vi "STEPkgDriver_LINC_Server.vi"() -> ()   [LabVIEW 2018, in "STEPkgDriver_LINC.lvlib"]
uses:
  STEPkgDriver_LINC.lvlib
  LINC/LINC.lvclass
  LINC/LINC Server Telemetry Prototype.ctl
  LINC/LINC Server Housekeeping.ctl
  LINC/LINC Server Command Prototype.vi
panel:
  in  "Manual Command String":string="SET_STRING with VAL \"Test Me\""
  in  "SET_VAR_STRING":string
  in  "command wait":u32
  out "Connected?":bool[](array[boolean])
  in  "Ports:":u16[](array[numeric])=[8000, 8001]
  in  "SET_U8_SCALED":dbl
  out "TEST_PACKET":T1={"COUNTER"=0, "NUMBER"=0.0, "STRING"="0000000000", "BOOLEAN"=FALSE, "ENUM"=enum."ENUM_ONE", "RING"=0, "ARRAY_U32"=[], "U8_SCALED"=0} {"U8_SCALED" format="%.3f"; "RING" items=["RING_ONE"=0, "RING_TWO"=1, "RING_THREE"=2, "RING_FOUR"=4]}
  in  "SET_ARRAY_U32":u32[](array[numeric])
  out "TELEMETRY:":string
  in  "SET_ERROR":bool
  in  "ERROR":errorcluster
  in  "SET_RING":u16(ring) items=["RING_ONE"=0, "RING_TWO"=1, "RING_THREE"=2, "RING_FOUR"=4]
  in  "SET_ENUM":enum16{"ENUM_ONE", "ENUM_TWO", "ENUM_THREE"}(ring)
  in  "SET_BOOLEAN":bool
  in  "SET_ALL":bool
  in  "SET_ALL":T2 {"RING" items=["RING_ONE"=0, "RING_TWO"=1, "RING_THREE"=2, "RING_FOUR"=4]}
  in  "SET_STRING":string
  in  "SET_NUMBER":dbl
  in  "COUNTER_INC":bool
  in  "COUNTER_RESET":bool
  in  "close":bool
  # "Manual Commands (Not available on RT):"
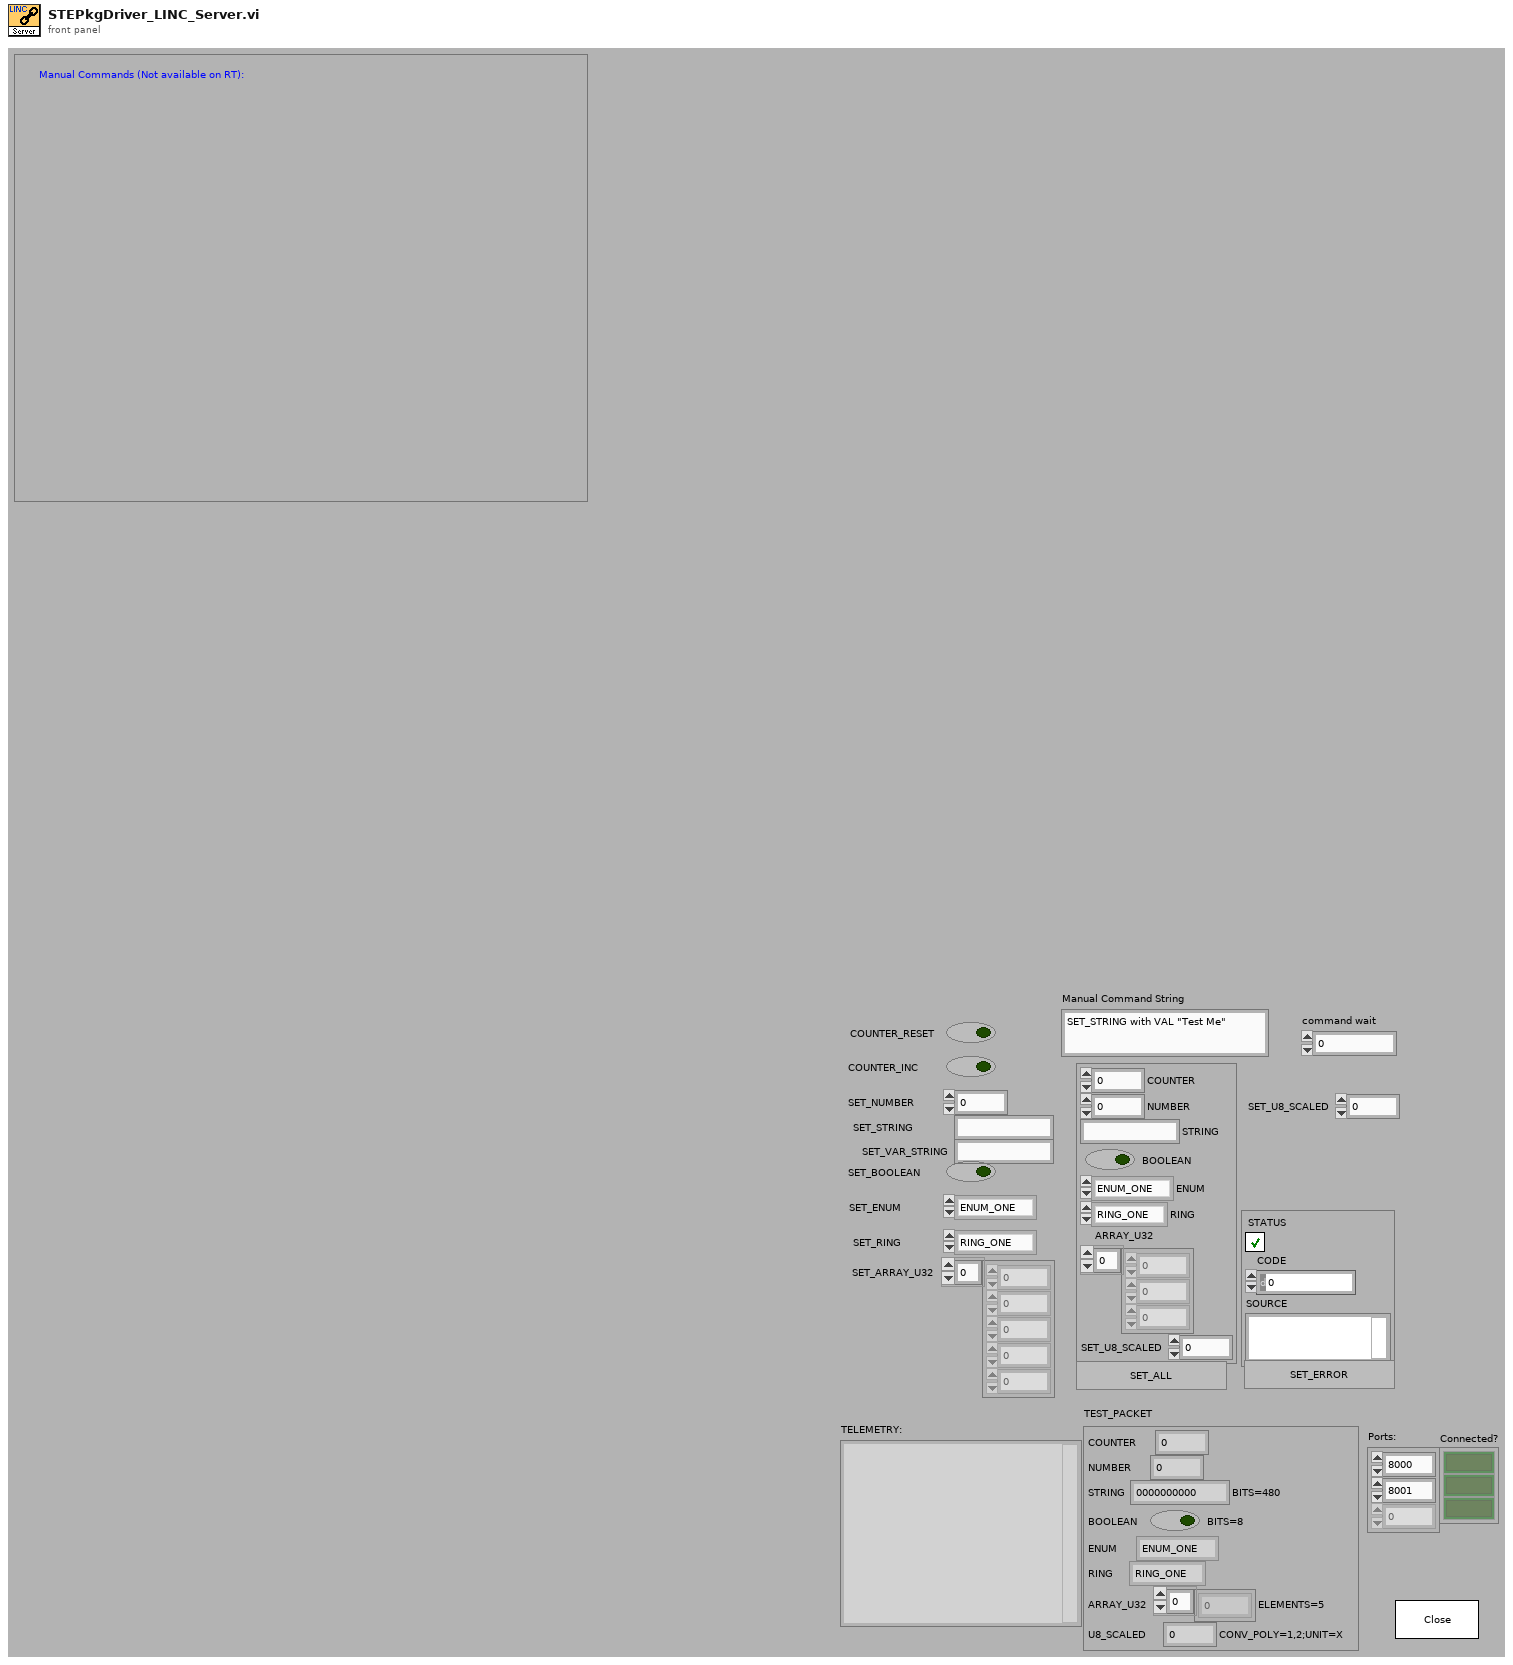
[diagram p1: front panel]
types:
  T1 = typedef "STEPkgDriver_LINC.lvlib/LINC Server Telemetry Prototype.ctl" = cluster{"COUNTER":u32, "NUMBER":dbl, "STRING":string, "BOOLEAN":bool, "ENUM":enum8{"ENUM_ONE", "ENUM_TWO", "ENUM_THREE"}, "RING":u8, "ARRAY_U32":u32[], "U8_SCALED":u8}
  T2 = cluster{"COUNTER":u32, "NUMBER":dbl, "STRING":string, "BOOLEAN":bool, "ENUM":enum16{"ENUM_ONE", "ENUM_TWO", "ENUM_THREE"}, "RING":u16, "ARRAY_U32":u32[], "SET_U8_SCALED":u8}
  T3 = typedef "STEPkgDriver_LINC.lvlib/LINC Server Housekeeping.ctl" = cluster{"TEST_PACKET":T1, "HANDSHAKING":bool}
  T4 = enum16{"initialize", "CMD", "TLM", "ERROR", "close"}
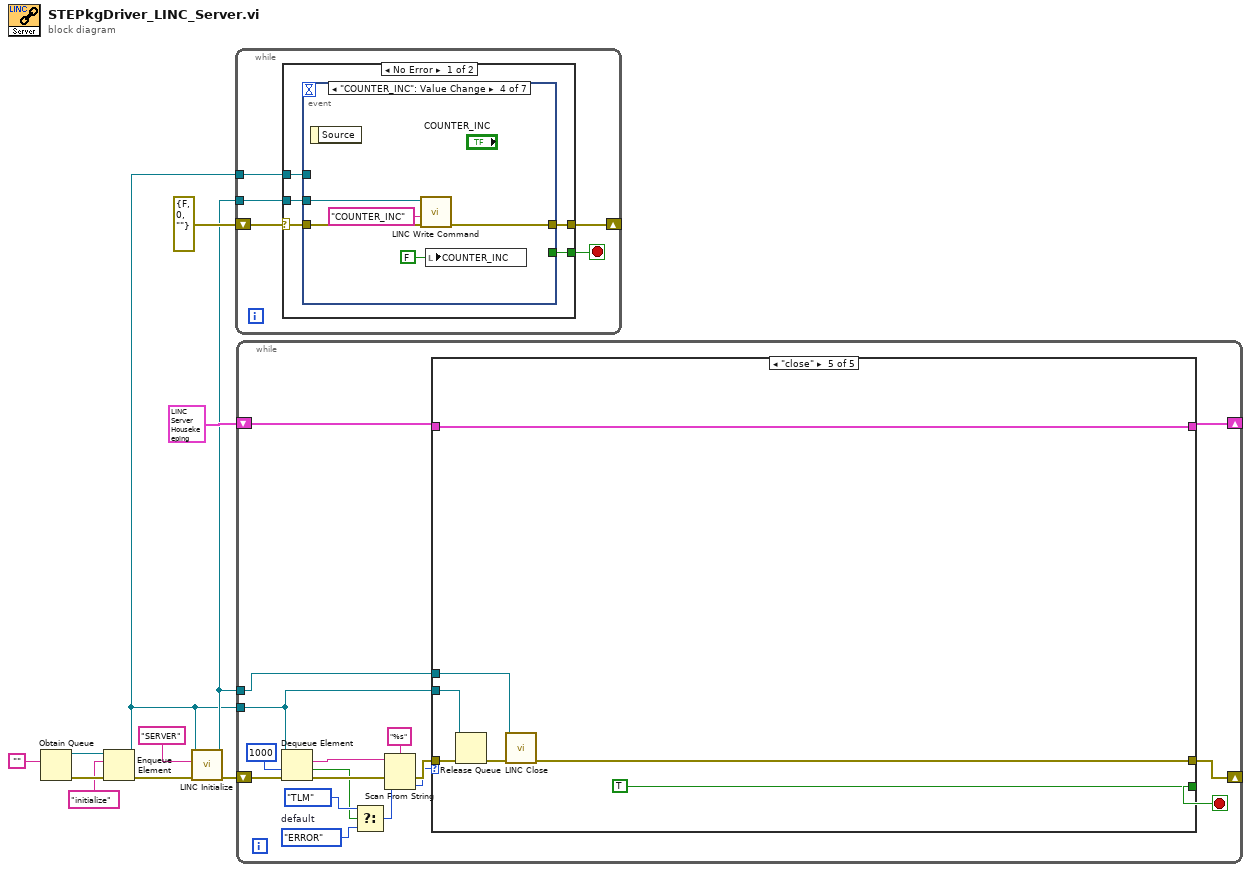
[diagram p0: block diagram]
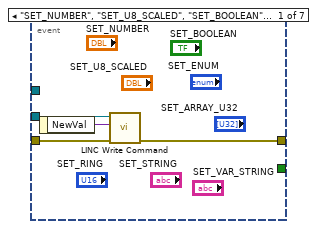
[diagram p2: hidden frame]
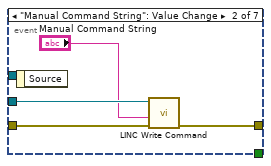
[diagram p3: hidden frame]
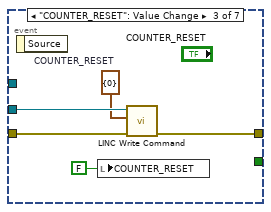
[diagram p4: hidden frame]
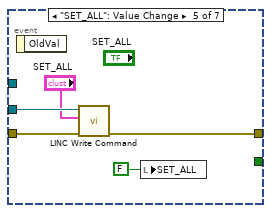
[diagram p5: hidden frame]
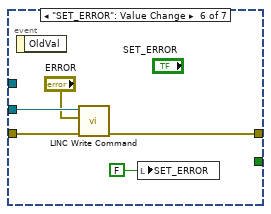
[diagram p6: hidden frame]
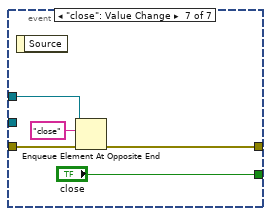
[diagram p7: hidden frame]
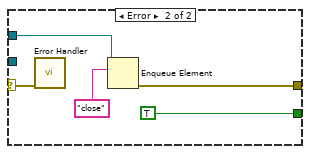
[diagram p8: hidden frame]
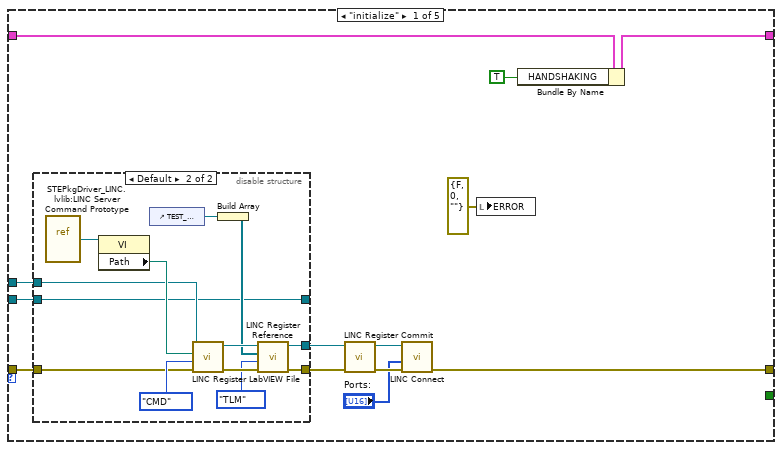
[diagram p9: hidden frame]
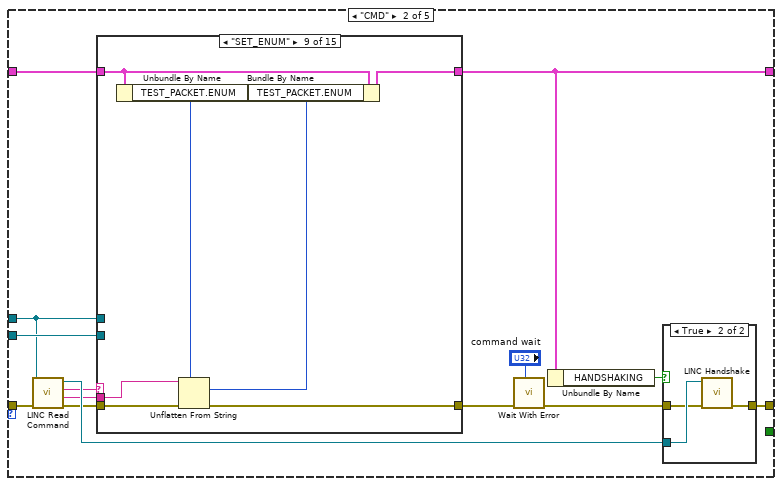
[diagram p11: hidden frame]
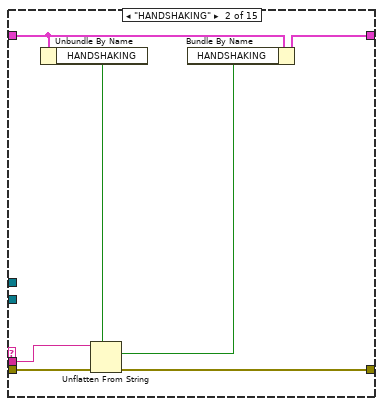
[diagram p14: hidden frame]
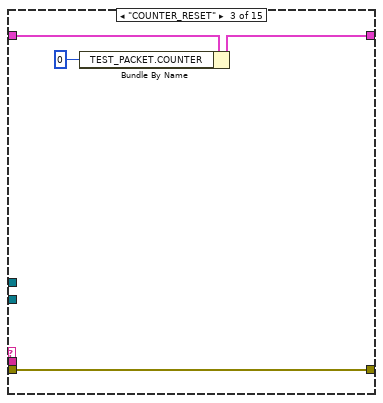
[diagram p15: hidden frame]
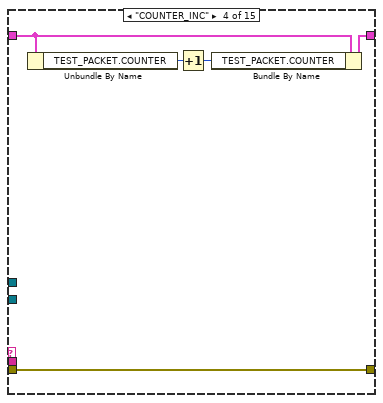
[diagram p16: hidden frame]
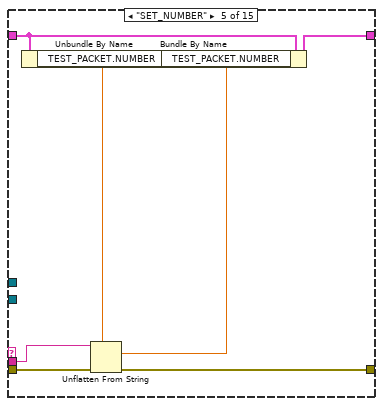
[diagram p17: hidden frame]
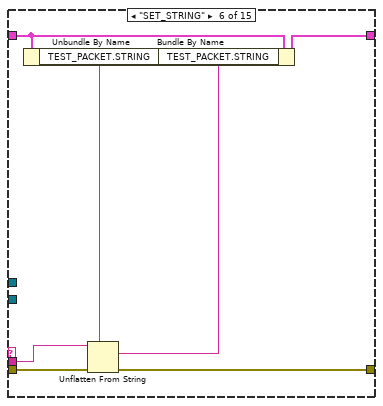
[diagram p18: hidden frame]
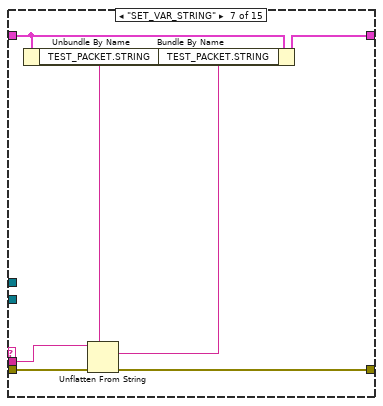
[diagram p19: hidden frame]
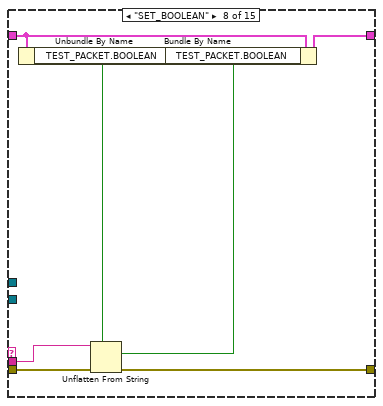
[diagram p20: hidden frame]
diagram:
  n1 = Obtain Queue(element data type="") -> (queue out=w9:refnum<queue>, error out=w10:errorcluster)  [unwired: 3 in, 2 out]
  n2 = Enqueue Element(queue=w9, element="initialize", error in (no error)=w10) -> (queue out=w1:refnum<queue>, error out=w7:errorcluster)  [unwired: 1 in, 1 out]
  n3 = call "LINC Initialize.vi"("error in (no error)"=w7, "target name"="SERVER", "application queue"=w1) -> ("error out"=w5:errorcluster, "LINC session"=w3:refnum<class "LINC.lvclass">)  [unwired: 3 in, 4 out]
  n4 = while {
    shift-right: [w14] -> _
    shift-left: errorcluster {"status"=FALSE, "code"=0, "source"=""} ("error out") -> [w16]
    tunnel: w3 -> [w13]
    tunnel: w1 -> [w12]
    stop <- w15 stop-if-true
    n5 = case shown="No Error" w16 {
      selector: w16 -> [w20 w58]
      tunnel: [w19 TRUE] -> w15
      tunnel: [w21 w56] -> w14
      tunnel: w13 -> [w18 _]
      tunnel: w12 -> [w17 w55]
      frame No Error {
        n6 = event shown="[3] \"COUNTER_INC\": Value Change" {
          selector: _ -> [_ _ _ _ _ _ _]
          dyn-events: _ -> [_ _ _ _ _ _ _]
          timeout: _ -> [_ _ _ _ _ _ _]
          tunnel: [w24 w27 w33 w38 w43 w48 w51] -> w21
          tunnel: w20 -> [w25 w29 w34 w39 w44 w49 w52]
          tunnel: [_ _ _ _ _ _ "close"] -> w19
          tunnel: w18 -> [w23 w28 w32 w37 w42 w47 _]
          tunnel: w17 -> [_ _ _ _ _ _ w50]
          event "SET_NUMBER", "SET_U8_SCALED", "SET_BOOLEAN", "SET_RING", "SET_ENUM", "SET_STRING", "SET_ARRAY_U32", "SET_VAR_STRING": Value Change {
            n7 = event-data() -> ("NewVal"=w22:variant)  [unwired: 1 out]
            n8 = call "LINC Write Command.vi"("error in (no error)"=w25, "packet"=w22, "LINC session"=w23) -> ("error out"=w24:errorcluster)  [unwired: 5 in, 3 out]
          }
          event "Manual Command String": Value Change {
            n9 = event-data() -> ()  [unwired: 2 out]
            n10 = call "LINC Write Command.vi"("error in (no error)"=w29, "string command"="Manual Command String", "LINC session"=w28) -> ("error out"=w27:errorcluster)  [unwired: 5 in, 3 out]
          }
          event "COUNTER_RESET": Value Change {
            w31 = cluster{"DUMMY":u8} {"DUMMY"=0}  # COUNTER_RESET
            n11 = event-data() -> ()  [unwired: 2 out]
            n12 = local write "COUNTER_RESET"(FALSE ("COUNTER_RESET")) -> ()
            n13 = call "LINC Write Command.vi"("error in (no error)"=w34, "packet"=w31, "LINC session"=w32) -> ("error out"=w33:errorcluster)  [unwired: 5 in, 3 out]
          }
          event "COUNTER_INC": Value Change {
            n14 = event-data() -> ()  [unwired: 2 out]
            n15 = call "LINC Write Command.vi"("error in (no error)"=w39, "string command"="COUNTER_INC", "LINC session"=w37) -> ("error out"=w38:errorcluster)  [unwired: 5 in, 3 out]
            n16 = local write "COUNTER_INC"(FALSE ("COUNTER_INC")) -> ()
          }
          event "SET_ALL": Value Change {
            n17 = event-data() -> ()  [unwired: 2 out]
            n18 = call "LINC Write Command.vi"("error in (no error)"=w44, "packet"="SET_ALL", "LINC session"=w42) -> ("error out"=w43:errorcluster)  [unwired: 5 in, 3 out]
            n19 = local write "SET_ALL"(FALSE ("SET_ALL")) -> ()
          }
          event "SET_ERROR": Value Change {
            n20 = event-data() -> ()  [unwired: 2 out]
            n21 = call "LINC Write Command.vi"("error in (no error)"=w49, "packet"="ERROR", "LINC session"=w47) -> ("error out"=w48:errorcluster)  [unwired: 5 in, 3 out]
            n22 = local write "SET_ERROR"(FALSE ("SET_ERROR")) -> ()
          }
          event "close": Value Change {
            n23 = event-data() -> ()  [unwired: 2 out]
            n24 = Enqueue Element At Opposite End(queue=w50, element="close", error in (no error)=w52) -> (error out=w51:errorcluster)  [unwired: 3 out]
          }
        }
      }
      frame Error {
        n25 = call "Error Handler.vi"("error in (no error)"=w58) -> ()  [unwired: 9 in, 2 out]
        n26 = Enqueue Element(queue=w55, element="close") -> (error out=w56:errorcluster)  [unwired: 2 in, 2 out]
      }
    }
  }
  n27 = while {
    shift-left: w5 -> [w70]
    shift-right: [w76] -> _
    tunnel: w1 -> [w69]
    shift-right: [w67] -> _
    shift-left: T3 {"TEST_PACKET"={"COUNTER"=0, "NUMBER"=0.0, "STRING"="", "BOOLEAN"=FALSE, "ENUM"=enum."ENUM_ONE", "RING"=0, "ARRAY_U32"=[], "U8_SCALED"=0}, "HANDSHAKING"=FALSE} -> [w68]
    tunnel: w3 -> [w65]
    stop <- w71 stop-if-true
    w62 = T4."ERROR"  # default
    n28 = Dequeue Element(queue=w69, timeout in ms (-1)=1000, error in (no error)=w70) -> (element=w66:string, timed out?=w60:bool, error out=w74:errorcluster)  [unwired: 1 out]
    n29 = Select(t=T4."TLM", s=w60, f=w62) -> (s? t:f=w61:T4)
    n30 = Scan From String(format string="%s", input string=w66, error in=w74, default 1=w61) -> (error out=w73:errorcluster, output 1=w72:T4)  [unwired: 1 in, 2 out]
    n31 = case shown="\"close\"" w72 {
      tunnel: w73 -> [w81 w114 w231 w240 w246]
      tunnel: [w82 w113 w218 _ w242] -> w76
      tunnel: [_ _ _ _ TRUE] -> w71
      tunnel: w69 -> [w77 w112 _ _ w247]
      tunnel: w68 -> [w88 w115 w230 w241 w245]
      tunnel: [w89 w111 w230 w241 w245] -> w67
      tunnel: w65 -> [w80 w109 w221 w239 w243]
      frame "initialize" {
        n32 = disable-structure shown="Default" {
          disable-tunnel: [w90 w105] -> w87
          disable-tunnel: [w91 w104] -> w86
          disable-tunnel: w81 -> [w90 w95]
          disable-tunnel: w80 -> [w91 w94]
          disable-tunnel: w77 -> [w92 w93]
          disable-tunnel: [w92 w93] -> _
          frame condition #0 {
            # "Dynamic registration is not avaliable on RT.  FTP SERVER_CMD.txt and SERVER_TLM.txt to above folder."
          }
          frame condition #1 (active) {
            n33 = vi-ref "STEPkgDriver_LINC.lvlib:LINC Server Command Prototype.vi"() -> (w97:refnum<vi>)
            n34 = property class="VI"(reference=w97) -> ("Path"=w96:path)  [unwired: 1 in, 2 out]
            n35 = control-ref of="TEST_PACKET"() -> (w101:refnum<vi>)
            n36 = call "LINC Register LabVIEW File.vi"("error in (no error)"=w95, "type (CMD)"=enum16{"CMD", "TLM", "CMD_HDR", "TLM_HDR"}."CMD", "prototype path"=w96, "LINC session"=w94) -> ("error out"=w103:errorcluster, "dup LINC session"=w102:refnum<class "LINC.lvclass">)  [unwired: 6 in]
            n37 = Build Array(w101) -> (w100:refnum<vi>[])
            n38 = call "LINC Register Reference.vi"("error in (no error)"=w103, "type (CMD)"=enum16{"CMD", "TLM", "CMD_HDR", "TLM_HDR"}."TLM", "controls"=w100, "LINC session"=w102) -> ("error out"=w105:errorcluster, "dup LINC session"=w104:refnum<class "LINC.lvclass">)  [unwired: 6 in]
          }
        }
        n39 = call "LINC Register Commit.vi"("error in (no error)"=w87, "LINC session"=w86) -> ("error out"=w84:errorcluster, "dup LINC session"=w83:refnum<class "LINC.lvclass">)  [unwired: 1 in, 7 out]
        n40 = call "LINC Connect.vi"("error in (no error)"=w84, "ports"="Ports:", "LINC session"=w83) -> ("error out"=w82:errorcluster)  [unwired: 7 in, 1 out]
        n41 = local write "ERROR"(errorcluster {"STATUS"=FALSE, "CODE"=0, "SOURCE"=""} ("ERROR")) -> ()
        n42 = Bundle By Name(cluster=w88, "HANDSHAKING"=TRUE) -> (w89:T3)
      }
      frame "CMD" {
        n43 = call "LINC Read Command.vi"("error in (no error)"=w114, "LINC session"=w109) -> ("error out"=w117:errorcluster, "cmd data"=w118:string, "cmd name"=w116:string, "dup LINC session"=w119:refnum<class "LINC.lvclass">)  [unwired: 2 in, 4 out]
        n44 = case shown="\"SET_ENUM\"" w116 {
          tunnel: w117 -> [w124 w129 w134 w140 w145 w152 w159 w166 w173 w180 w188 w195 w202 w208 w214]
          tunnel: w115 -> [w125 w127 w136 w139 w142 w150 w157 w164 w171 w178 w185 w192 w199 w209 w216]
          tunnel: [w125 w132 w135 w141 w148 w155 w162 w169 w176 w183 w190 w197 w204 w209 w216] -> w111
          tunnel: [w124 w128 w134 w140 w144 w151 w158 w165 w172 w179 w187 w194 w201 w205 w213] -> w108
          tunnel: w112 -> [_ _ _ _ _ _ _ _ _ _ _ _ _ _ w212]
          tunnel: w118 -> [_ w131 _ _ w147 w154 w161 w168 w175 w182 w189 w196 w203 w211 _]
          tunnel: w109 -> [_ _ _ _ _ _ _ _ _ _ _ _ _ _ _]
          frame Default {
          }
          frame "HANDSHAKING" {
            n45 = Unbundle By Name(w127) -> ("HANDSHAKING"=w126:bool)
            n46 = Unflatten From String(type=w126, binary string=w131, error in (no error)=w129) -> (value=w130:bool, error out=w128:errorcluster)  [unwired: 2 in, 1 out]
            n47 = Bundle By Name(cluster=w127, "HANDSHAKING"=w130) -> (w132:T3)
          }
          frame "COUNTER_RESET" {
            n48 = Bundle By Name(cluster=w136, "TEST_PACKET.COUNTER"=u32 0 ("counter")) -> (w135:T3)
          }
          frame "COUNTER_INC" {
            n49 = Unbundle By Name(w139) -> ("TEST_PACKET.COUNTER"=w138:u32)
            n50 = Increment(x=w138) -> (x+1=w137:u32)
            n51 = Bundle By Name(cluster=w139, "TEST_PACKET.COUNTER"=w137) -> (w141:T3)
          }
          frame "SET_NUMBER" {
            n52 = Unbundle By Name(w142) -> ("TEST_PACKET.NUMBER"=w143:dbl)
            n53 = Unflatten From String(type=w143, binary string=w147, error in (no error)=w145) -> (value=w146:dbl, error out=w144:errorcluster)  [unwired: 2 in, 1 out]
            n54 = Bundle By Name(cluster=w142, "TEST_PACKET.NUMBER"=w146) -> (w148:T3)
          }
          frame "SET_STRING" {
            n55 = Unbundle By Name(w150) -> ("TEST_PACKET.STRING"=w149:string)
            n56 = Unflatten From String(type=w149, binary string=w154, error in (no error)=w152) -> (value=w153:string, error out=w151:errorcluster)  [unwired: 2 in, 1 out]
            n57 = Bundle By Name(cluster=w150, "TEST_PACKET.STRING"=w153) -> (w155:T3)
          }
          frame "SET_VAR_STRING" {
            n58 = Unbundle By Name(w157) -> ("TEST_PACKET.STRING"=w156:string)
            n59 = Unflatten From String(type=w156, binary string=w161, error in (no error)=w159) -> (value=w160:string, error out=w158:errorcluster)  [unwired: 2 in, 1 out]
            n60 = Bundle By Name(cluster=w157, "TEST_PACKET.STRING"=w160) -> (w162:T3)
          }
          frame "SET_BOOLEAN" {
            n61 = Unbundle By Name(w164) -> ("TEST_PACKET.BOOLEAN"=w163:bool)
            n62 = Unflatten From String(type=w163, binary string=w168, error in (no error)=w166) -> (value=w167:bool, error out=w165:errorcluster)  [unwired: 2 in, 1 out]
            n63 = Bundle By Name(cluster=w164, "TEST_PACKET.BOOLEAN"=w167) -> (w169:T3)
          }
          frame "SET_ENUM" {
            n64 = Unbundle By Name(w171) -> ("TEST_PACKET.ENUM"=w170:enum8{"ENUM_ONE", "ENUM_TWO", "ENUM_THREE"})
            n65 = Unflatten From String(type=w170, binary string=w175, error in (no error)=w173) -> (value=w174:enum8{"ENUM_ONE", "ENUM_TWO", "ENUM_THREE"}, error out=w172:errorcluster)  [unwired: 2 in, 1 out]
            n66 = Bundle By Name(cluster=w171, "TEST_PACKET.ENUM"=w174) -> (w176:T3)
          }
          frame "SET_RING" {
            n67 = Unbundle By Name(w178) -> ("TEST_PACKET.RING"=w177:u8)
            n68 = Unflatten From String(type=w177, binary string=w182, error in (no error)=w180) -> (value=w181:u8, error out=w179:errorcluster)  [unwired: 2 in, 1 out]
            n69 = Bundle By Name(cluster=w178, "TEST_PACKET.RING"=w181) -> (w183:T3)
          }
          frame "SET_ALL" {
            n70 = Unbundle By Name(w185) -> ("TEST_PACKET"=w184:T1)
            n71 = Unflatten From String(type=w184, binary string=w189, error in (no error)=w188) -> (value=w186:T1, error out=w187:errorcluster)  [unwired: 2 in, 1 out]
            n72 = Bundle By Name(cluster=w185, "TEST_PACKET"=w186) -> (w190:T3)
          }
          frame "SET_ARRAY_U32" {
            n73 = Unbundle By Name(w192) -> ("TEST_PACKET.ARRAY_U32"=w191:u32[])
            n74 = Unflatten From String(type=w191, binary string=w196, error in (no error)=w195) -> (value=w193:u32[], error out=w194:errorcluster)  [unwired: 2 in, 1 out]
            n75 = Bundle By Name(cluster=w192, "TEST_PACKET.ARRAY_U32"=w193) -> (w197:T3)
          }
          frame "SET_U8_SCALED" {
            n76 = Unbundle By Name(w199) -> ("TEST_PACKET.U8_SCALED"=w198:u8)
            n77 = Unflatten From String(type=w198, binary string=w203, error in (no error)=w202) -> (value=w200:u8, error out=w201:errorcluster)  [unwired: 2 in, 1 out]
            n78 = Bundle By Name(cluster=w199, "TEST_PACKET.U8_SCALED"=w200) -> (w204:T3)
          }
          frame "ERROR" {
            n79 = Unflatten From String(type=errorcluster {"STATUS"=FALSE, "CODE"=0, "SOURCE"=""} ("ERROR"), binary string=w211, error in (no error)=w208) -> (value=w207:errorcluster, error out=w206:errorcluster)  [unwired: 2 in, 1 out]
            n80 = Merge Errors(w206, w207) -> (w205:errorcluster)
          }
          frame "QUIT" {
            n81 = Enqueue Element At Opposite End(queue=w212, element="close", error in (no error)=w214) -> (error out=w213:errorcluster)  [unwired: 3 out]
          }
        }
        n82 = call "Wait With Error.vi"("milliseconds to wait"="command wait", "error in (no error)"=w108) -> ("error out"=w107:errorcluster)  [unwired: 9 in]
        n83 = Unbundle By Name(w111) -> ("HANDSHAKING"=w110:bool)
        n84 = case shown="True" w110 {
          tunnel: w119 -> [_ w123]
          tunnel: w107 -> [w120 w122]
          tunnel: [w120 w121] -> w113
          frame False {
          }
          frame True {
            n85 = call "LINC Handshake.vi"("error in (no error)"=w122, "LINC session"=w123) -> ("error out"=w121:errorcluster)  [unwired: 8 in, 1 out]
          }
        }
      }
      frame "TLM" {
        n86 = Unbundle By Name(w230) -> ("TEST_PACKET"=w223:T1)
        "TEST_PACKET" <- w223
        n87 = call "LINC Write Telemetry.vi"("error in (no error)"=w231, "packet"=w223, "LINC session"=w221) -> ("error out"=w229:errorcluster, "dup LINC session"=w228:refnum<class "LINC.lvclass">)  [unwired: 4 in, 3 out]
        n88 = call "LINC Read Telemetry.vi"("mode (single)"=enum16{"single", "packet", "all"}."all", "error in (no error)"=w229, "LINC session"=w228) -> ("error out"=w220:errorcluster, "item values"=w226:string[], "item names"=w227:string[], "dup LINC session"=w219:refnum<class "LINC.lvclass">)  [unwired: 4 in, 1 out]
        n89 = for {
          tunnel: w227 -> [w237] mode=indexing
          tunnel: w226 -> [w236] mode=indexing
          shift-right: [w232] -> w224
          shift-left: "" -> [w234]
          n90 = Format Into String(format string="%s: %s\n", w237, w236) -> (resulting string=w233:string)  [unwired: 2 in, 1 out]
          n91 = Concatenate Strings(w234, w233) -> (w232:string)
        }
        "TELEMETRY:" <- w224
        n92 = call "LINC Get Connection Status.vi"("error in (no error)"=w220, "LINC session"=w219) -> ("error out"=w218:errorcluster, "connected"=→"Connected?":bool[])  [unwired: 7 in, 1 out]
      }
      frame "ERROR" {
        n93 = call "LINC Error.vi"("error in (no error)"=w240, "LINC session"=w239) -> ("error out"=w238:errorcluster)  [unwired: 8 in, 1 out]
        n94 = local write "ERROR"(w238) -> ()
      }
      frame "close" {
        n95 = Release Queue(queue=w247, error in (no error)=w246) -> (error out=w244:errorcluster)  [unwired: 3 out]
        n96 = call "LINC Close.vi"("error in (no error)"=w244, "LINC session"=w243) -> ("error out"=w242:errorcluster)  [unwired: 9 out]
      }
    }
  }
